vi "lib Degrees Arcmin Arcsec to Degrees decimal.vi"(8 "error in (no error)":errorcluster, 11 "Declination":T1) -> (0 "error out":errorcluster, 3 "Angle":dbl format="%#.8g")   [LabVIEW 2024]
uses:
  Telescope/Telescope cluster Declination.ctl
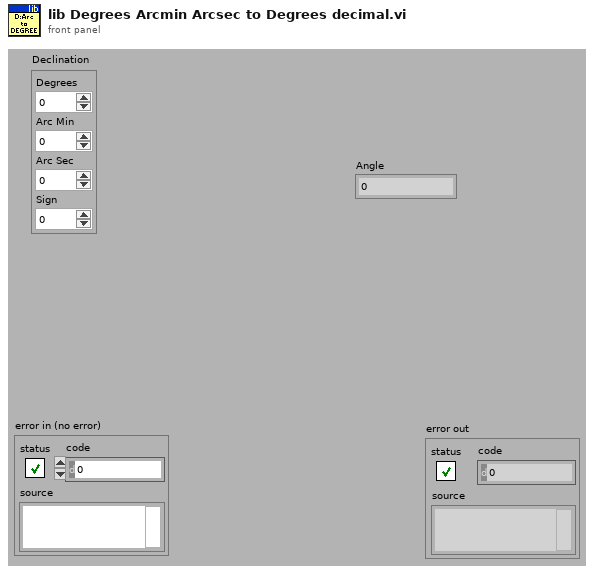
[diagram p1: front panel]
types:
  T1 = typedef "Telescope cluster Declination.ctl" = cluster{"Degrees":dbl, "Arc Min":dbl, "Arc Sec":dbl, "Sign":dbl}
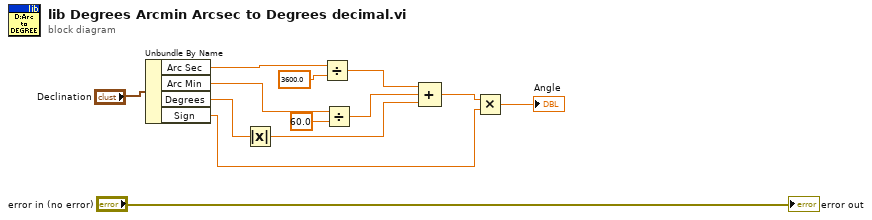
[diagram p0: block diagram]
diagram:
  n1 = Unbundle By Name("Declination") -> ("Arc Sec"=w10:dbl, "Arc Min"=w9:dbl, "Degrees"=w5:dbl, "Sign"=w3:dbl)
  n2 = Absolute Value(x=w5) -> (abs(x)=w6:dbl)
  n3 = Divide(x=w10, y=3600.0) -> (x/y=w8:dbl)
  n4 = Divide(x=w9, y=60.0) -> (x/y=w7:dbl)
  n5 = Compound Arithmetic op=ADD(w8, w7, w6) -> (w4:dbl)
  n6 = Multiply(x=w4, y=w3) -> (x*y=→"Angle":dbl)
  "error out" <- "error in (no error)"
